vi "Add Info Log.vi"(8 "error in (no error)":errorcluster, 10 "Info":string, 11 "Server in":refnum<class "Server.lvclass">) -> (0 "error out":errorcluster, 3 "Server out":refnum<class "Server.lvclass">)   [LabVIEW 2020, in "HTTP Server.lvlib" / "Server.lvclass"]
uses:
  Server.lvclass
  Access Log Entry.ctl
  Server.lvclass/Server.ctl
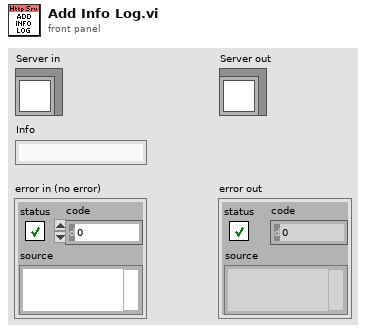
[diagram p1: front panel]
types:
  T1 = typedef "HTTP Server.lvlib/Server.lvclass/Access Log Entry.ctl" = cluster{"Time Stamp":timestamp, "Client":string, "Code":u16, "Info":string}
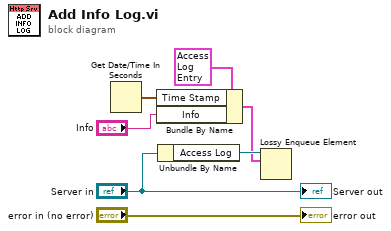
[diagram p0: block diagram]
diagram:
  n1 = Get Date/Time In Seconds() -> (seconds since 1Jan1904=w2:timestamp)
  n2 = Bundle By Name(cluster=T1 {"Time Stamp"=timestamp(0 s since 1904-01-01), "Client"="", "Code"=0, "Info"=""} ("element"), "Time Stamp"=w2, "Info"="Info") -> (w3:T1)
  n3 = Unbundle By Name("Server in") -> ("Access Log"=w5:refnum<queue>)
  n4 = Lossy Enqueue Element(queue=w5, element=w3) -> ()  [unwired: 1 in, 4 out]
  "error out" <- "error in (no error)"
  "Server out" <- "Server in"
